vi "updateValues.vi"(6 "units":i16=2, 7 "device and axis array":string[](array[string]), 8 "error in (no error)":errorcluster, 9 "channel index":i32, 10 "microstep sizes array":dbl[](array[numeric]), 11 "VISA resource name":refnum<visa-resource-name>) -> (0 "error out":errorcluster, 3 "VISA resource name out":refnum<visa-resource-name>)   [LabVIEW 2020, in "ZaberASeries.lvclass"]
uses:
  ZaberASeries.lvclass
  Zaber A Series.lvlib
panel:
  out "Response String Array":string[](array[string])
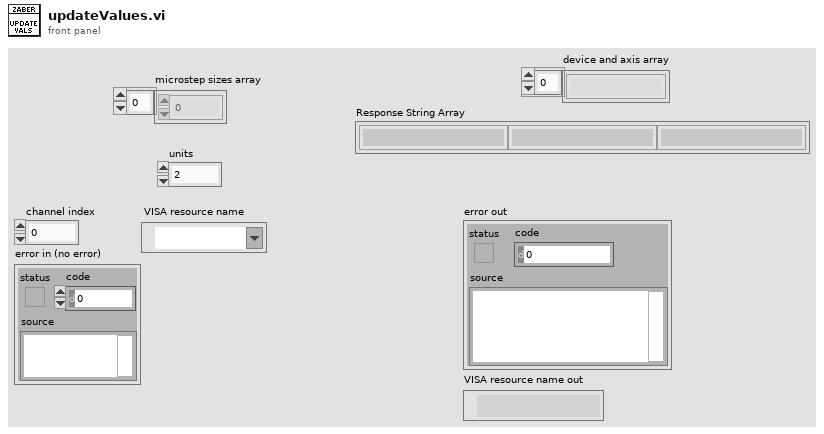
[diagram p1: front panel]
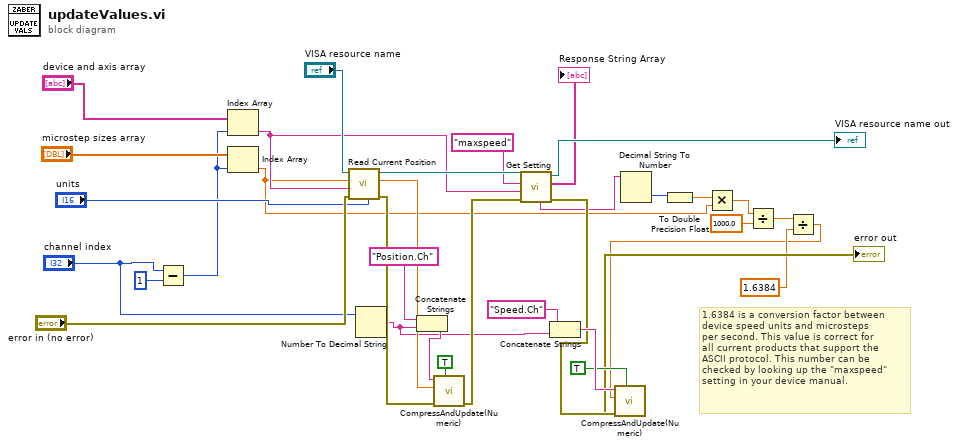
[diagram p0: block diagram]
diagram:
  # "1.6384 is a conversion factor between \ndevice speed units and microsteps \nper second. This value is correct for\nall current products that support the\nASCII protocol. This number can be \nchecked by looking up the \"maxspeed\"\nsetting in your device manual."
  n1 = Subtract(x="channel index", y=1) -> (x-y=w23:i32)
  n2 = Index Array(array="device and axis array", index=w23) -> (element=w18:string)
  n3 = Index Array(array="microstep sizes array", index=w23) -> (element=w7:dbl)
  n4 = call "Read Current Position.vi"("Units (0: microsteps)"="units", "error in (no error)"="error in (no error)", "Device and Axis"=w18, "Microstep Size (0)"=w7, "VISA resource name"="VISA resource name") -> ("error out"=w29:errorcluster, "Position"=w28:dbl, "VISA resource name out"=w21:refnum<visa-resource-name>)  [unwired: 4 in]
  n5 = Number To Decimal String(number="channel index") -> (decimal integer string=w13:string)  [unwired: 1 in]
  n6 = Concatenate Strings("Position.Ch" ("command or variable name"), w13) -> (w34:string)
  n7 = call "CompressAndUpdate(Numeric).vi"("force CVT update (false)"=TRUE, "error in"=w29, "Numeric"=w28, "command or variable name"=w34) -> ("error out"=w17:errorcluster)  [unwired: 7 in]
  n8 = call "Get Setting.vi"("error in (no error)"=w17, "Device and Axis"=w18, "Setting"="maxspeed", "VISA resource name"=w21) -> ("error out"=w12:errorcluster, "Response String Array"=→"Response String Array":string[], "VISA resource name out"=→"VISA resource name out":refnum<visa-resource-name>, "First Response Data"=w10:string)  [unwired: 2 in, 2 out]
  n9 = Concatenate Strings("Speed.Ch" ("command or variable name"), w13) -> (w16:string)
  n10 = Decimal String To Number(string=w10) -> (number=w9:i32)  [unwired: 2 in, 1 out]
  n11 = To Double Precision Float(number=w9) -> (double precision float=w6:dbl)
  n12 = Multiply(x=w6, y=w7) -> (x*y=w5:dbl)
  n13 = Divide(x=w5, y=1000.0) -> (x/y=w3:dbl)
  n14 = Divide(x=w3, y=1.6384 ("Speed Constant (1.6384)")) -> (x/y=w1:dbl)
  n15 = call "CompressAndUpdate(Numeric).vi"("force CVT update (false)"=TRUE, "error in"=w12, "Numeric"=w1, "command or variable name"=w16) -> ("error out"=→"error out":errorcluster)  [unwired: 7 in]
